vi "Export_txt.vi"(8 "error in (no error)":errorcluster, 11 "Analysis List ref":refnum<vi>) -> (0 "error out":errorcluster)   [LabVIEW 2015]
doc: "Exports the selected samples into a text file"
uses:
  global_variables.vi
  Classes/AnalysisList/AnalysisList.lvclass
  Classes/AnalysisListItems/AnalysisListItems.lvclass
  MSControl/Classes/Analysis/Analysis.lvclass
panel:
  out "Slide":u16(slide) max=18 step=1 scale=0.0..17.0
  # "Exporting Data"
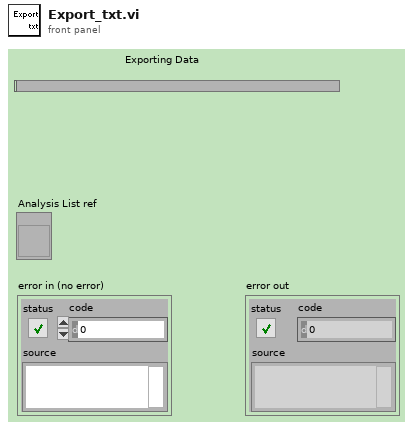
[diagram p1: front panel]
types:
  T1 = enum16{"open", "replace", "create", "open or create", "replace or create", "replace or create with confirmation"}
  T2 = typedef "ExtrapolationResultsArray.ctl" = string[][]
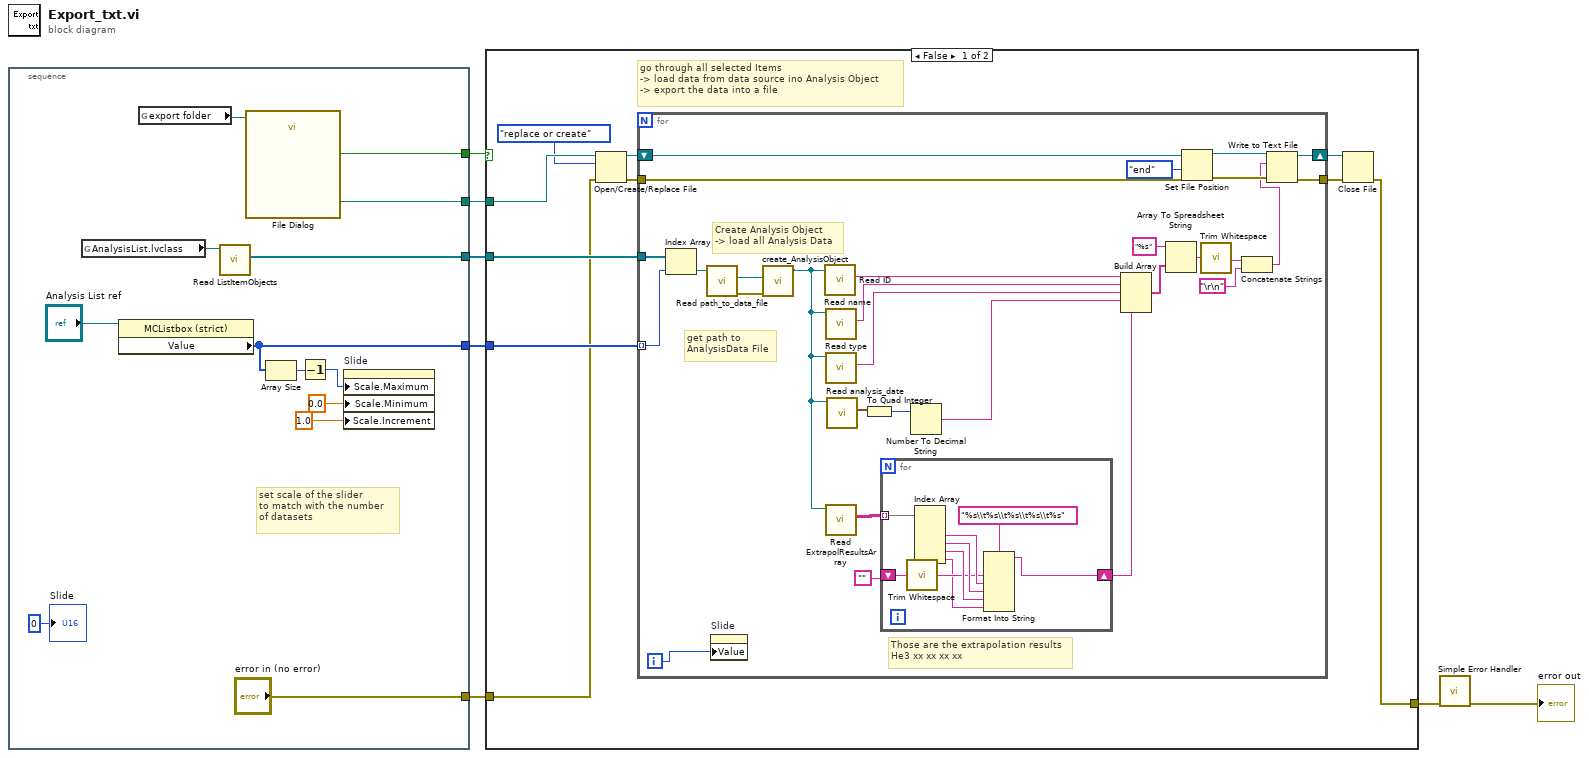
[diagram p0: block diagram]
diagram:
  n1 = stacked-sequence {
    tunnel: [w17] -> w7
    tunnel: [w18] -> w6
    tunnel: [w13] -> w5
    tunnel: [w12] -> w4
    tunnel: ["error in (no error)"] -> w3
    frame #0 {
      # "set scale of the slider\nto match with the number\nof datasets"
      n2 = global read "global_variables.vi" "AnalysisList.lvclass"() -> (w19:refnum<class "AnalysisList.lvclass">)
      n3 = property class="MCListbox (strict)"(reference="Analysis List ref") -> ("Value"=w17:i32[])  [unwired: 1 in, 2 out]
      n4 = global read "global_variables.vi" "export folder"() -> (w14:path)
      n5 = call-dynamic "Read ListItemObjects.vi"("AnalysisList in"=w19) -> ("AnalysisObjects"=w18:refnum<class "AnalysisListItems.lvclass">[])  [unwired: 8 in, 2 out]
      n6 = call "File Dialog"("start path"=w14) -> ("selected path"=w12:path, "cancelled"=w13:bool)  [unwired: 11 in, 2 out]
      n7 = Array Size(array=w17) -> (size(s)=w9:i32)
      n8 = Decrement(x=w9) -> (x-1=w8:i32)
      n9 = property on="Slide" class="Slide (strict)"("Scale.Maximum"=w8, "Scale.Minimum"=0.0 ("Data Entry Limits:Minimum"), "Scale.Increment"=1.0 ("Data Entry Limits:Increment")) -> ()  [unwired: 2 in, 2 out]
      "Slide" <- u8 0 ("Slide")
    }
  }
  n10 = case shown="False" w5 {
    tunnel: w7 -> [w30 _]
    tunnel: w6 -> [w29 _]
    tunnel: w4 -> [w28 _]
    tunnel: w3 -> [w21 w69]
    tunnel: [w22 w69] -> w2
    frame False {
      # "go through all selected Items\n-> load data from data source ino Analysis Object\n-> export the data into a file"
      n11 = Open/Create/Replace File(file path (use dialog)=w28, error in=w21, operation (0:open)=T1."replace or create") -> (refnum out=w27:refnum<file>, error out=w25:errorcluster)  [unwired: 3 in, 1 out]
      n12 = for {
        tunnel: w30 -> [w58] mode=indexing
        tunnel: w29 -> [w59]
        tunnel: w25 -> [w36]
        shift-right: [w40] -> w24
        shift-left: w27 -> [w38]
        tunnel: [w39] -> w23
        i -> [w41]
        # "Create Analysis Object\n-> load all Analysis Data"
        # "get path to\nAnalysisData File"
        # "Those are the extrapolation results\nHe3 xx xx xx xx"
        n13 = Index Array(array=w59, index=w58) -> (element=w43:refnum<class "AnalysisListItems.lvclass">)
        n14 = call-dynamic "Read path_to_data_file.vi"("AnalysisListItems in"=w43) -> ("error out"=w45:errorcluster, "path_to_data_file"=w44:path)  [unwired: 8 in, 1 out]
        n15 = property on="Slide" class="Slide (strict)"("Value"=w41) -> ()  [unwired: 2 in, 2 out]
        n16 = call "create_AnalysisObject.vi"("error in (no error)"=w45, "FilePath"=w44) -> ("Analysis out"=w42:refnum<class "Analysis.lvclass">)  [unwired: 8 in, 1 out]
        n17 = call-dynamic "Read ID.vi"("Analysis in"=w42) -> ("ID"=w57:string)  [unwired: 8 in, 2 out]
        n18 = call-dynamic "Read name.vi"("Analysis in"=w42) -> ("name"=w56:string)  [unwired: 8 in, 2 out]
        n19 = call-dynamic "Read type.vi"("Analysis in"=w42) -> ("type"=w55:string)  [unwired: 8 in, 2 out]
        n20 = call-dynamic "Read ExtrapolResultsArray.vi"("Analysis in"=w42) -> ("ExtrapolResultsArray"=w54:T2)  [unwired: 8 in, 2 out]
        n21 = call-dynamic "Read analysis_date.vi"("Analysis in"=w42) -> ("analysis date"=w49:timestamp)  [unwired: 8 in, 2 out]
        n22 = To Quad Integer(1:w49) -> (0:w47:i64)
        n23 = for {
          tunnel: w54 -> [w63] mode=indexing
          shift-right: [w64] -> w48
          shift-left: "" -> [w62]
          n24 = call <vilib>:"Trim Whitespace.vi"("string"=w62) -> ("trimmed string"=w61:string)  [unwired: 1 in]
          n25 = Index Array(array=w63) -> (element #2=w68:string, element #3=w67:string, element #4=w66:string, element #5=w60:string)  [unwired: 5 in, 1 out]
          n26 = Format Into String(format string="%s\\t%s\\t%s\\t%s\\t%s", w61, w68, w67, w66, w60) -> (resulting string=w64:string)  [unwired: 2 in, 1 out]
        }
        n27 = Number To Decimal String(number=w47) -> (decimal integer string=w46:string)  [unwired: 1 in]
        n28 = Build Array(w57, w56, w55, w46, w48) -> (w52:string[])
        n29 = Array To Spreadsheet String(array=w52, 3:"%s" ("format string")) -> (spreadsheet string=w50:string)  [unwired: 1 in]
        n30 = Set File Position(refnum=w38, from (0:start)=enum16{"start", "end", "current"}."end", error in=w36) -> (refnum out=w37:refnum<file>, error out=w35:errorcluster)  [unwired: 1 in]
        n31 = call <vilib>:"Trim Whitespace.vi"("string"=w50) -> ("trimmed string"=w33:string)  [unwired: 1 in]
        n32 = Concatenate Strings(w33, "\r\n") -> (w31:string)
        n33 = Write to Text File(file (use dialog)=w37, text=w31, error in=w35) -> (refnum out=w40:refnum<file>, error out=w39:errorcluster)  [unwired: 1 in, 1 out]
      }
      n34 = Close File(refnum=w24, error in=w23) -> (error out=w22:errorcluster)  [unwired: 1 out]
    }
    frame True {
      # "Dialog canceled, don't save data"
    }
  }
  n35 = call <vilib>:"Simple Error Handler.vi"("error in (no error)"=w2) -> ("error out"=→"error out":errorcluster)  [unwired: 4 in, 4 out]
